vi "Parse Path Array indexes.vi"(9 "error in (no error)":errorcluster, 11 "Path with leading Array element":string) -> (1 "error out":errorcluster, 2 "Indexes (empty means use all)":i32[](array[numeric]), 3 "Rest or Path":string, 4 "Max Index to parse":i32)   [LabVIEW 2019, in "JSONtext.lvlib"]
uses:
  JSONtext.lvlib
  Parsing State.ctl
  JSON Value Type.ctl
  Advance past Line Ending.vi
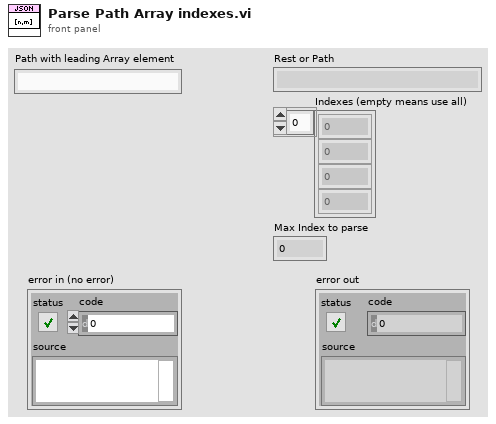
[diagram p1: front panel]
types:
  T1 = typedef "JSONtext.lvlib/Parsing State.ctl" = enum16{"Parser Error", "Object", "Array", "String", "Number/Other", "Leading Whitespace", "Object end", "Array end", "Value end"}
  T2 = typedef "JSONtext.lvlib/JSON Value Type.ctl" = enum16{"Not a JSON Value", "JSON Object", "JSON Array", "String", "Number", "true", "false", "null"}
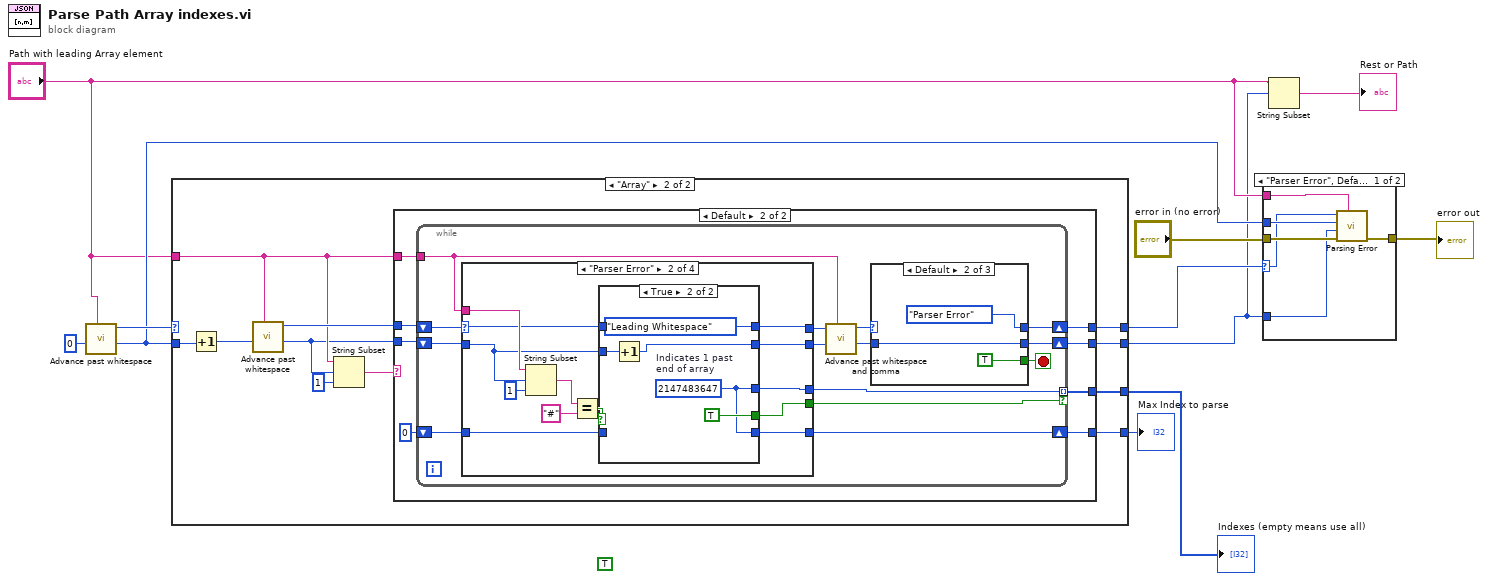
[diagram p0: block diagram]
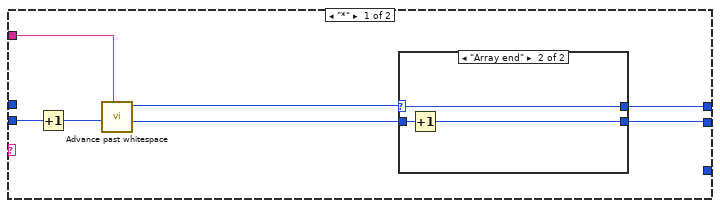
[diagram p4: hidden frame]
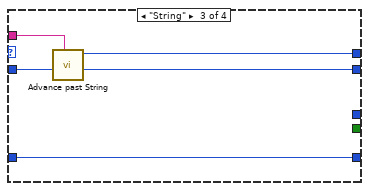
[diagram p8: hidden frame]
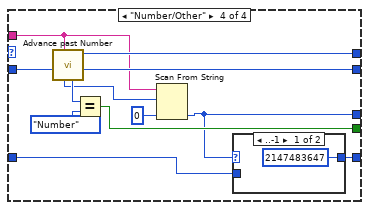
[diagram p9: hidden frame]
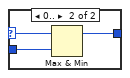
[diagram p10: hidden frame]
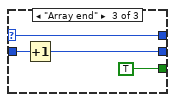
[diagram p12: hidden frame]
diagram:
  (unwired) TRUE
  n1 = call "Advance past whitespace.vi"("JSON"="Path with leading Array element", "Offset"=0) -> ("Offset of first non-whitespace"=w7:i32, "Parser State"=w11:T1)  [unwired: 7 in, 1 out]
  n2 = case shown="\"Array\"" w11 {
    selector: w11 -> [w12 _]
    tunnel: w7 -> [w13 w24]
    tunnel: "Path with leading Array element" -> [_ w21]
    tunnel: [_ w17] -> w6
    tunnel: [w13 w16] -> w3
    tunnel: [w12 w15] -> w8
    tunnel: [_ w14] -> w1
    frame "Parser Error", Default {
    }
    frame "Array" {
      n3 = Increment(x=w24) -> (x+1=w22:i32)
      n4 = call "Advance past whitespace.vi"("JSON"=w21, "Offset"=w22) -> ("Offset of first non-whitespace"=w20:i32, "Parser State"=w23:T1)  [unwired: 7 in, 1 out]
      n5 = String Subset(string=w21, offset (0)=w20, length (rest)=1 ("length (rest)")) -> (substring=w18:string)
      n6 = case shown="Default" w18 {
        tunnel: w23 -> [_ w44]
        tunnel: w21 -> [w25 w43]
        tunnel: w20 -> [w31 w42]
        tunnel: [_ w41] -> w17
        tunnel: [w27 w40] -> w16
        tunnel: [w26 w39] -> w15
        tunnel: [_ w37] -> w14
        frame "*" {
          n7 = Increment(x=w31) -> (x+1=w30:i32)
          n8 = call "Advance past whitespace.vi"("JSON"=w25, "Offset"=w30) -> ("Offset of first non-whitespace"=w28:i32, "Parser State"=w29:T1)  [unwired: 7 in, 1 out]
          n9 = case shown="\"Array end\"" w29 {
            selector: w29 -> [w33 w34]
            tunnel: w28 -> [w32 w36]
            tunnel: [w32 w35] -> w27
            tunnel: [w33 w34] -> w26
            frame "Parser Error", Default {
            }
            frame "Array end" {
              n10 = Increment(x=w36) -> (x+1=w35:i32)
            }
          }
        }
        frame Default {
          n11 = while {
            tunnel: w43 -> [w51]
            shift-right: [w56] -> w40
            shift-left: w42 -> [w49]
            shift-right: [w52] -> w39
            shift-left: w44 -> [w50]
            tunnel: [w48] -> w41 mode=indexing if=w47
            shift-right: [w46] -> w37
            shift-left: 0 -> [w45]
            stop <- w55 stop-if-true
            n12 = case shown="\"Parser Error\"" w50 {
              selector: w50 -> [w61 w64 _ _]
              tunnel: w49 -> [w60 w66 w86 w97]
              tunnel: [w61 w67 w87 w99] -> w54
              tunnel: [w60 w65 w84 w98] -> w53
              tunnel: w51 -> [_ w74 w85 w93]
              tunnel: [_ w69 _ w90] -> w48
              tunnel: [_ w68 _ w94] -> w47
              tunnel: [w59 w63 w83 w89] -> w46
              tunnel: w45 -> [w59 w62 w83 w88]
              frame Default {
              }
              frame "Parser Error" {
                n13 = String Subset(string=w74, offset (0)=w66, length (rest)=1 ("length (rest)")) -> (substring=w72:string)
                n14 = Equal?(x=w72, y="#") -> (x = y?=w70:bool)
                n15 = case shown="True" w70 {
                  tunnel: [_ w78] -> w69
                  tunnel: [_ TRUE] -> w68
                  tunnel: [w77 Parsing_State."Leading Whitespace" ("Parser State")] -> w67
                  tunnel: w66 -> [w76 w80]
                  tunnel: [w76 w79] -> w65
                  tunnel: w64 -> [w77 _]
                  tunnel: [w75 w78] -> w63
                  tunnel: w62 -> [w75 _]
                  frame False {
                  }
                  frame True {
                    w78 = 2147483647  # Indicates 1 past end of array
                    n16 = Increment(x=w80) -> (x+1=w79:i32)
                  }
                }
              }
              frame "String" {
                n17 = call "Advance past String.vi"("JSON"=w85, "Offset"=w86) -> ("Offset past match"=w84:i32, "State"=w87:T1)  [unwired: 7 in, 1 out]
              }
              frame "Number/Other" {
                n18 = call "Advance past Number.vi"("JSON"=w93, "Offset (0)"=w97) -> ("Offset past match"=w98:i32, "Parser State"=w99:T1, "JSON Value Type"=w96:T2, "Value start out"=w92:i32)  [unwired: 6 in]
                n19 = Equal?(x=w96, y=JSON_Value_Type."Number") -> (x = y?=w94:bool)
                n20 = Scan From String(input string=w93, initial scan location=w92, default 1=0) -> (output 1=w90:i32)  [unwired: 2 in, 3 out]
                n21 = case shown="..-1" w90 {
                  selector: w90 -> [_ w103]
                  tunnel: [2147483647 w102] -> w89
                  tunnel: w88 -> [_ w101]
                  frame ..-1 {
                  }
                  frame 0.. {
                    n22 = Max & Min(x=w103, y=w101) -> (max(x,y)=w102:i32)  [unwired: 1 out]
                  }
                }
              }
            }
            n23 = call "Advance past whitespace and comma.vi"("JSON"=w51, "Offset"=w53, "State in"=w54) -> ("Offset past match"=w58:i32, "State"=w57:T1)  [unwired: 6 in, 1 out]
            n24 = case shown="Default" w57 {
              selector: w57 -> [w104 _ w109]
              tunnel: [_ TRUE TRUE] -> w55
              tunnel: w58 -> [w105 w107 w111]
              tunnel: [w105 w107 w110] -> w56
              tunnel: [w104 Parsing_State."Parser Error" w109] -> w52
              frame "Number/Other" {
              }
              frame Default {
              }
              frame "Array end" {
                n25 = Increment(x=w111) -> (x+1=w110:i32)
              }
            }
          }
        }
      }
    }
  }
  "Indexes (empty means use all)" <- w6
  "Max Index to parse" <- w1
  n26 = case shown="\"Parser Error\", Default" w8 {
    selector: w8 -> [w113 _]
    tunnel: "Path with leading Array element" -> [w118 _]
    tunnel: "error in (no error)" -> [w117 w119]
    tunnel: [w116 w119] -> w9
    tunnel: w7 -> [w115 _]
    tunnel: w3 -> [w114 _]
    frame "Parser Error", Default {
      n27 = call "Parsing Error.vi"("JSON"=w118, "error in (no error)"=w117, "Offset past match"=w114, "Value start"=w115, "State"=w113) -> ("error out"=w116:errorcluster)  [unwired: 6 in]
    }
    frame "Array end" {
    }
  }
  "error out" <- w9
  n28 = String Subset(string="Path with leading Array element", offset (0)=w3) -> (substring=→"Rest or Path":string)  [unwired: 1 in]
